vi "Targets 2 Command Data.vi"(10 "Target  Inputs":T1[](array[typedef])) -> (2 "LBCB 2 Command Data":T3, 3 "LBCB 1 Command Data":T3)   [LabVIEW 2009]
uses:
  Target Data.ctl
  Data Access Objects/Metadata/LBCB Space.ctl
  Target.ctl
  Data Access Objects/Metadata/LBCB Number.ctl
  Apps/App Status Actions.ctl
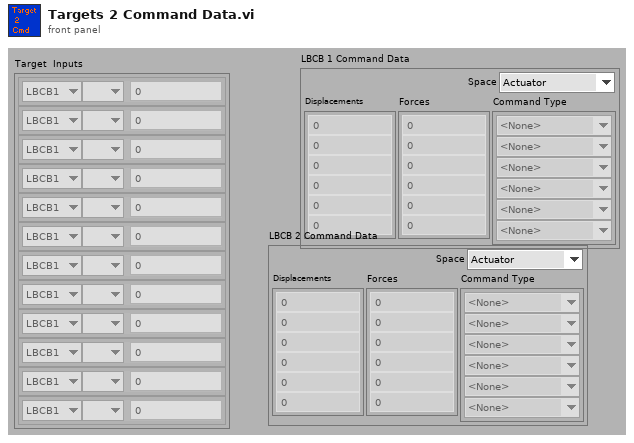
[diagram p1: front panel]
types:
  T1 = typedef "Target.ctl" = cluster{"LBCB Number":T2, "DOF Vectors":enum16{" ", "Dx", "Dy", "Dz", "Rx", "Ry", "Rz", "Fx", "Fy", "Fz", "Mx", "My", "Mz"}, "Amount":dbl}
  T2 = typedef "LBCB Number.ctl" = enum16{"LBCB1", "LBCB2"}
  T3 = typedef "Target Data.ctl" = cluster{"Displacements":dbl[], "Command Type":enum16{"<None>", "Displacement", "Force"}[], "Forces":dbl[], "Space":T4}
  T4 = typedef "LBCB Space.ctl" = enum16{"Actuator", "Cartesian"}
  T5 = typedef "App Status Actions.ctl" = enum16{"Init", "Get Status", "Running", "Control", "Autobalanced", "Data Acquisition", "Set App State", "DAQ Started", "Set LBCB State", "Set All", "Set Cont Logging", "Set Step Logging", "Set MM Logging", "Set Volt Logging", "Set Cart Type", "Set DAQ Link", "Set NTCP Link"}
  T6 = typedef "App Status.ctl" = cluster{"Running":bool, "Controlling L2":bool, "Autobalance L2":bool, "Data Acquisition":bool, " App State":T7, "DAQ Started":bool, "LBCB 1 State":T8, "LBCB 2 State":T8, "Controlling L1":bool, "Autobalance L1":bool, "Cartesian Type":bool, "Continuous Logging":bool, "Step Logging":bool, "Voltage Logging":bool, "Mixed Mode Logging":bool, "DAQ Link":bool, "NTCP Link ":bool}
  T7 = typedef "AppStates.ctl" = enum16{"Starting OM", "Initializing Displays", "Setting up Archiving", "Setting Up DAQ Channels", "Start DAQ", "DAQ Starting", "Controlling LBCBs", "Stopping OM"}
  T8 = typedef "Lbcb Control Loop States.ctl" = enum16{"Idle", "Load Last Command", "Start Autobalancing", "Autobalancing", "Control Loop Initialized", "Control Enabled"}
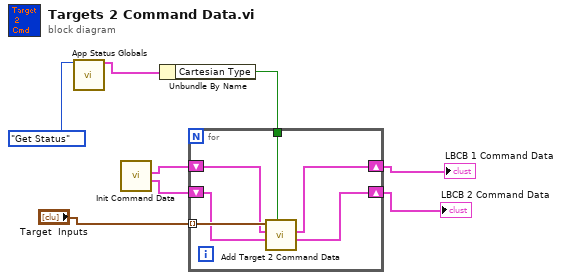
[diagram p0: block diagram]
diagram:
  n1 = call "App Status Globals.vi"("App Status Actions"=App_Status_Actions."Get Status") -> ("App Status Out"=w3:T6)  [unwired: 5 in, 9 out]
  n2 = call "Init Command Data.vi"() -> ("LBCB 2 Command Data"=w6:T3, "LBCB 1 Command Data"=w7:T3)  [unwired: 10 out]
  n3 = Unbundle By Name(w3) -> ("Cartesian Type"=w2:bool)
  n4 = for {
    tunnel: "Target  Inputs" -> [w14] mode=indexing
    shift-right: [w11] -> w5
    shift-left: w7 -> [w12]
    shift-right: [w10] -> w4
    shift-left: w6 -> [w13]
    tunnel: w2 -> [w9]
    n5 = call "Add Target 2 Command Data.vi"("Cartesian Type"=w9, "LBCB 2 Command Data In"=w13, "LBCB 1 Command Data In"=w12, "Target"=w14) -> ("LBCB 2 Command Data Out"=w10:T3, "LBCB 1 Command Data Out"=w11:T3)  [unwired: 6 out]
  }
  "LBCB 1 Command Data" <- w5
  "LBCB 2 Command Data" <- w4
